vi "Get Help File Link.vi"(8 "error in (no error)":errorcluster, 11 "Files Installed":path[](array[path])) -> (0 "error out":errorcluster, 2 "Link Valid?":bool, 3 "Help File Link":string)   [LabVIEW 2015]
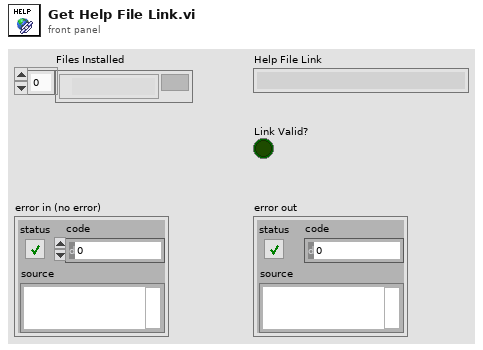
[diagram p1: front panel]
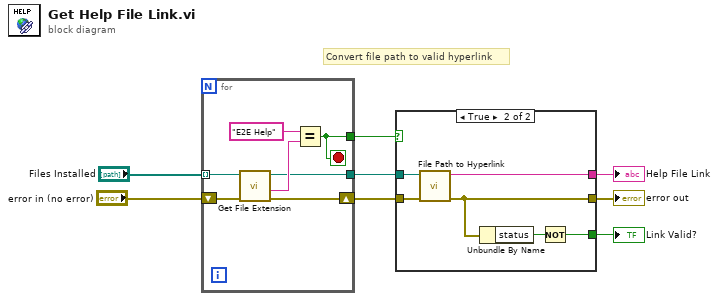
[diagram p0: block diagram]
diagram:
  # "Convert file path to valid hyperlink"
  n1 = for {
    tunnel: "Files Installed" -> [w15] mode=indexing
    shift-right: [w14] -> w7
    shift-left: "error in (no error)" -> [w13]
    tunnel: [w10] -> w5
    tunnel: [w9] -> w6
    stop <- w9 stop-if-true
    n2 = call <vilib>:"Get File Extension.vi"("error in (no error)"=w13, "file"=w15) -> ("error out"=w14:errorcluster, "filename without extension"=w12:string, "dup file"=w10:path)  [unwired: 5 in, 2 out]
    n3 = Equal?(x="E2E Help", y=w12) -> (x = y?=w9:bool)
  }
  n4 = case shown="True" w6 {
    tunnel: w7 -> [w16 w20]
    tunnel: w5 -> [_ w22]
    tunnel: [_ w21] -> w4
    tunnel: [_ w17] -> w2
    tunnel: [w16 w19] -> w1
    frame False {
    }
    frame True {
      n5 = call "File Path to Hyperlink.vi"("error in (no error)"=w20, "File Path"=w22) -> ("error out"=w19:errorcluster, "Hyperlink"=w21:string)  [unwired: 8 in]
      n6 = Unbundle By Name(w19) -> ("status"=w18:bool)
      n7 = Not(x=w18) -> (.not. x?=w17:bool)
    }
  }
  "Help File Link" <- w4
  "Link Valid?" <- w2
  "error out" <- w1
